vi "Prototype.vi"(8 "error in (no error)":errorcluster, 10 "Prototyper in":refnum<class "Prototyper.lvclass">, 11 "Scripter in":refnum<class "Message Scripter.lvclass">) -> (0 "error out":errorcluster, 2 "Prototyper out":refnum<class "Prototyper.lvclass">, 3 "Scripter out":refnum<class "Message Scripter.lvclass">)   [LabVIEW 2020, in "Message Maker.lvlib" / "Prototyper.lvclass"]
uses:
  Prototyper.lvclass
  Message Scripter/Message Scripter.lvclass
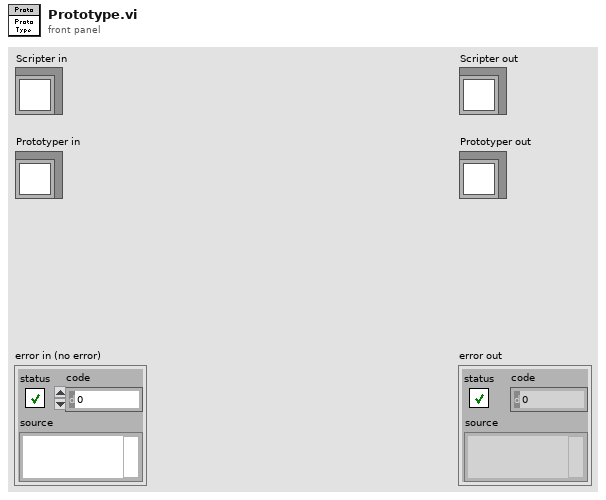
[diagram p1: front panel]
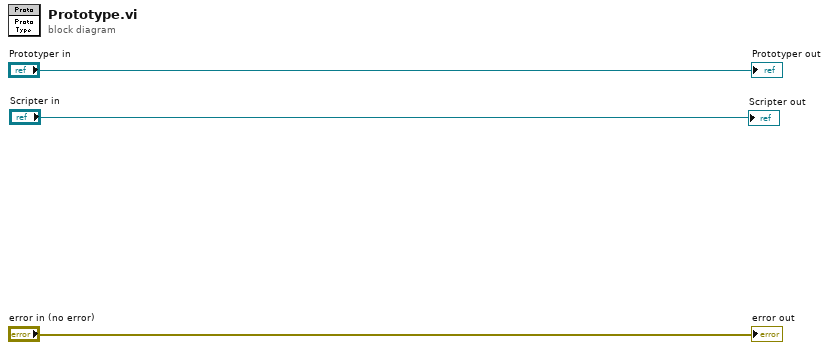
[diagram p0: block diagram]
diagram:
  "error out" <- "error in (no error)"
  "Prototyper out" <- "Prototyper in"
  "Scripter out" <- "Scripter in"
